vi "Read BMS Data.vi"(8 "error in (no error)":errorcluster, 11 "OrionBMS in":refnum<class "OrionBMSClass.lvclass">) -> (0 "error out":errorcluster, 2 "BMS Data":T1, 3 "OrionBMS out":refnum<class "OrionBMSClass.lvclass">)   [LabVIEW 2018, in "OrionBMSClass.lvclass"]
uses:
  OrionBMSClass.lvclass
  Type_Def/TypeDef_BMSDatas.ctl
  Type_Def/TypeDef_BMSStatuss.ctl
  OrionBMSClass.lvclass/OrionBMSClass.ctl
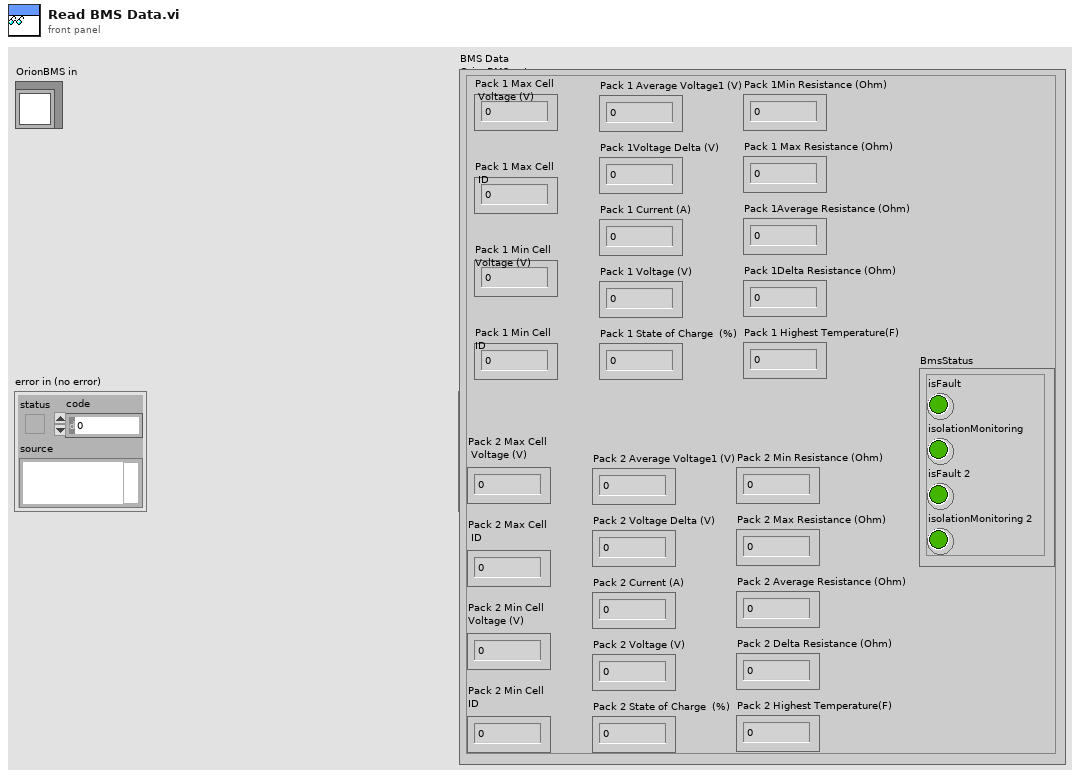
[diagram p1: front panel]
types:
  T1 = typedef "TypeDef_BMSDatas.ctl" = cluster{"Pack 1 Max Cell\n Voltage (V)":dbl, "Pack 1 Max Cell\n ID ":dbl, "Pack 1 Min Cell \nVoltage (V)":dbl, "Pack 1 Min Cell \nID ":dbl, "Pack 1 State of Charge  (%)":dbl, "Pack 1 Average Voltage1 (V)":dbl, "Pack 1Voltage Delta (V)":dbl, "Pack 1 Current (A)":dbl, "Pack 1 Voltage (V)":dbl, "Pack 1 Max Resistance (Ohm)":dbl, "Pack 1Min Resistance (Ohm)":dbl, "Pack 1Average Resistance (Ohm)":dbl, "Pack 1Delta Resistance (Ohm)":dbl, "Pack 1 Highest Temperature(F)":dbl, "BmsStatus":T2, "Pack 2 Max Cell\n Voltage (V) ":dbl, "Pack 2 Max Cell\n ID  ":dbl, "Pack 2 Min Cell \nVoltage (V) ":dbl, "Pack 2 Min Cell \nID  ":dbl, "Pack 2 Average Voltage1 (V)":dbl, "Pack 2 Voltage Delta (V) ":dbl, "Pack 2 Current (A)":dbl, "Pack 2 Voltage (V) ":dbl, "Pack 2 State of Charge  (%) ":dbl, "Pack 2 Max Resistance (Ohm) ":dbl, "Pack 2 Min Resistance (Ohm)":dbl, "Pack 2 Average Resistance (Ohm)":dbl, "Pack 2 Delta Resistance (Ohm) ":dbl, "Pack 2 Highest Temperature(F) ":dbl}
  T2 = typedef "TypeDef_BMSStatuss.ctl" = cluster{"isFault":bool, "isolationMonitoring":bool, "isFault 2":bool, "isolationMonitoring 2":bool}
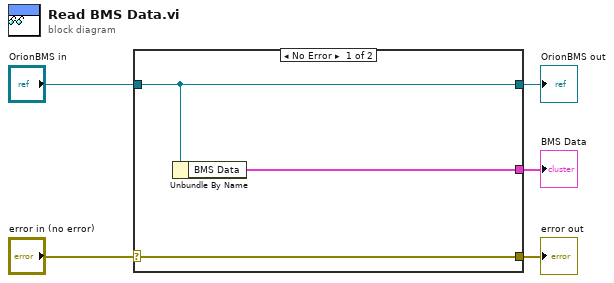
[diagram p0: block diagram]
diagram:
  n1 = case shown="No Error" "error in (no error)" {
    selector: "error in (no error)" -> [w8 w9]
    tunnel: [w8 w9] -> w4
    tunnel: [w7 w10] -> w2
    tunnel: "OrionBMS in" -> [w7 w10]
    tunnel: [w6 _] -> w1
    frame No Error {
      n2 = Unbundle By Name(w7) -> ("BMS Data"=w6:T1)
    }
    frame Error {
    }
  }
  "error out" <- w4
  "OrionBMS out" <- w2
  "BMS Data" <- w1
